vi "pH Setpoint Step Configuration.vi"(8 "error in (no error)":errorcluster, 10 "Parameters In":variant, 11 "Subpanel Queue In":refnum<queue>) -> (0 "error out":errorcluster, 2 "Parameters Out":variant)   [LabVIEW 2018]
doc: "Configuration control for the 'Set pH Setpoint' step."
panel:
  in  "pH Setpoint":dbl min=0.0 max=14.0
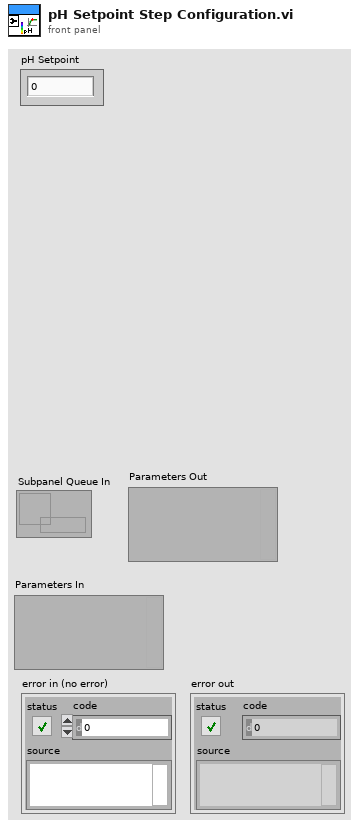
[diagram p1: front panel]
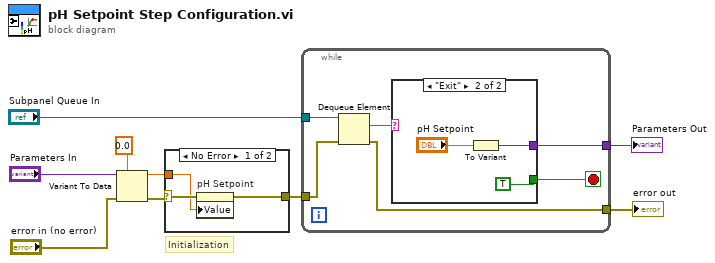
[diagram p0: block diagram]
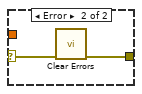
[diagram p2: hidden frame]
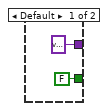
[diagram p3: hidden frame]
diagram:
  # "Initialization"
  n1 = Variant To Data(error in="error in (no error)", type=0.0 ("pH Setpoint"), Variant="Parameters In") -> (data=w4:dbl, error out=w5:errorcluster)
  n2 = case shown="No Error" w5 {
    selector: w5 -> [w12 w14]
    tunnel: w4 -> [w11 _]
    tunnel: [w10 w13] -> w3
    frame No Error {
      n3 = property on="pH Setpoint" class="DigNum (strict)"(error in=w12, "Value"=w11) -> (error out=w10:errorcluster)  [unwired: 1 in, 1 out]
    }
    frame Error {
      n4 = call <vilib>:"Clear Errors.vi"("error in (no error)"=w14) -> ("error out"=w13:errorcluster)  [unwired: 5 in, 1 out]
    }
  }
  n5 = while {
    tunnel: [w20] -> w9
    tunnel: "Subpanel Queue In" -> [w19]
    tunnel: w3 -> [w17]
    tunnel: [w15] -> w1
    stop <- w16 stop-if-true
    n6 = Dequeue Element(queue=w19, error in (no error)=w17) -> (element=w18:string, error out=w15:errorcluster)  [unwired: 1 in, 2 out]
    n7 = case shown="\"Exit\"" w18 {
      tunnel: [variant ("Variant") w25] -> w20
      tunnel: [FALSE TRUE] -> w16
      frame Default {
      }
      frame "Exit" {
        n8 = To Variant(anything="pH Setpoint") -> (Variant=w25:variant)
      }
    }
  }
  "Parameters Out" <- w9
  "error out" <- w1
